vi "init_dataframe.vi"(10 "data":string, 11 "command type":T1) -> (3 "DataFrame.lvclass":refnum<class "DataFrame.lvclass">)   [LabVIEW 2017, in "DataFrame.lvclass"]
uses:
  DataFrame.lvclass
  command_type.ctl
  DataFrame.lvclass/DataFrame.ctl
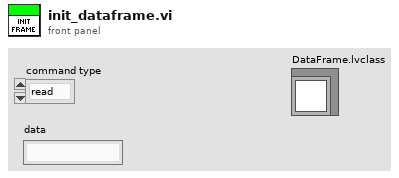
[diagram p1: front panel]
types:
  T1 = typedef "DataFrame.lvclass/command_type.ctl" = enum8{"read", "write"}
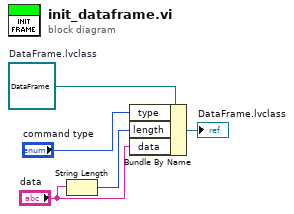
[diagram p0: block diagram]
diagram:
  w5 = refnum<class "DataFrame.lvclass"> refnum  # DataFrame.lvclass
  n1 = String Length(string="data") -> (length=w1:i32)
  n2 = Bundle By Name(cluster=w5, "type"="command type", "length"=w1, "data"="data") -> (→"DataFrame.lvclass":refnum<class "DataFrame.lvclass">)
